vi "VisionAnalysisUI.vi"(11 "FunctionNames":string[](array[string])) -> ()   [LabVIEW 2015]
uses:
  [Global]VisionAnalysis_DVR.vi
  VisionAnalysisFramework/PackedLibrary/VisionAnalysisFramework.lvlibp/VisionAnalysisFramework/Object/VisionAnalysisFramework.lvclass
panel:
  in  "index":i32
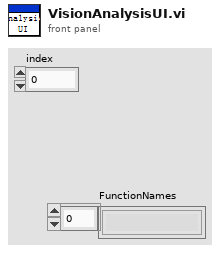
[diagram p1: front panel]
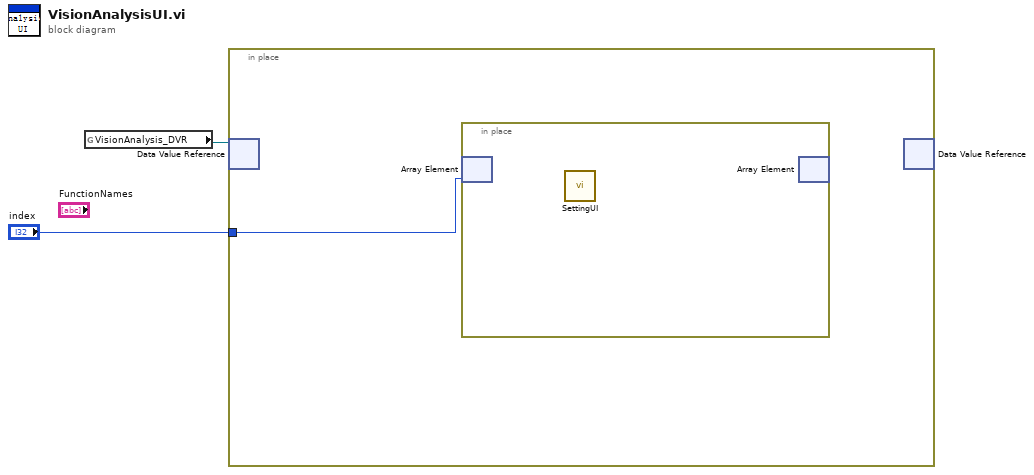
[diagram p0: block diagram]
diagram:
  n1 = global read "[Global]VisionAnalysis_DVR.vi" "VisionAnalysis_DVR"() -> (w3:refnum<data-value>)
  n2 = in-place {
    in-place-border: "index" -> [w4]
    n3 = in-place-dvr #1(w3) -> ()  [unwired: 2 out]
    n4 = in-place {
      n5 = in-place-array #2(w4) -> ()  [unwired: 1 in, 1 out]
      n6 = call-dynamic "SettingUI.vi"() -> ()  [unwired: 10 in, 2 out]
      n7 = in-place-array #2() -> ()  [unwired: 1 in, 2 out]
    }
    n8 = in-place-dvr #1() -> ()  [unwired: 1 in, 2 out]
  }
